vi "W&R(Know Size Without Check With Data).vi"(0 "VISA resource name in":refnum<visa-resource-name>, 5 "写入指令/数据":string, 7 "总字节数":u32, 9 "超时":u32=1000, 11 "error in":errorcluster) -> (4 "VISA resource name out":refnum<visa-resource-name>, 6 "读取缓冲区":string, 15 "error out":errorcluster)   [LabVIEW 2020]
uses:
  <vilib>/Instr/_visa.llb/VISA Set IO Buffer Mask.ctl
  <vilib>/Instr/_visa.llb/VISA Flush IO Buffer Mask.ctl
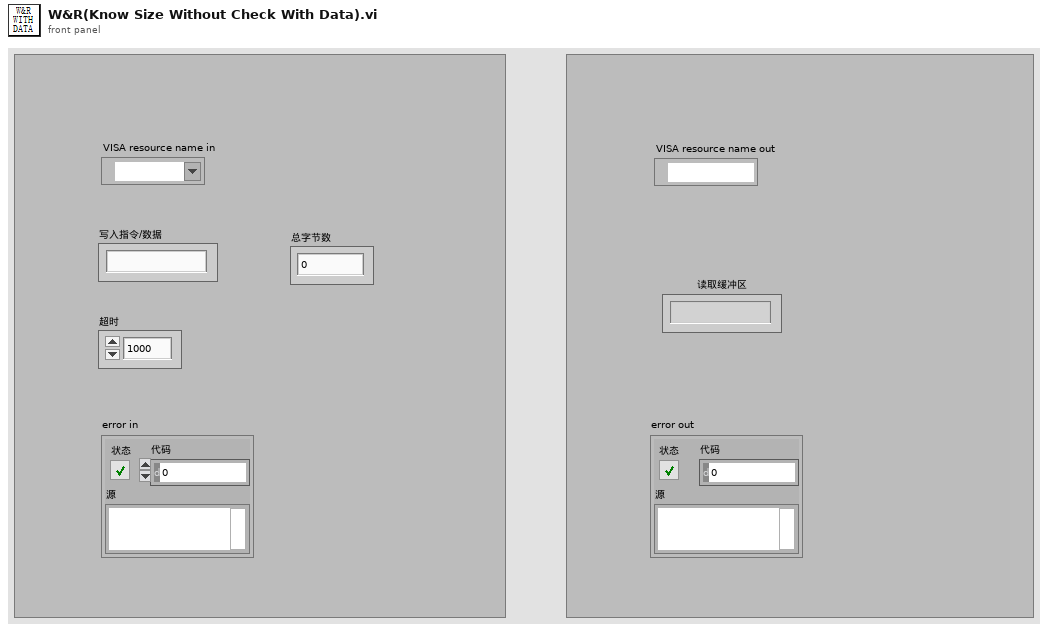
[diagram p1: front panel]
types:
  T1 = typedef "VISA Flush IO Buffer Mask.ctl" = u16
  T2 = typedef "VISA Set IO Buffer Mask.ctl" = u16
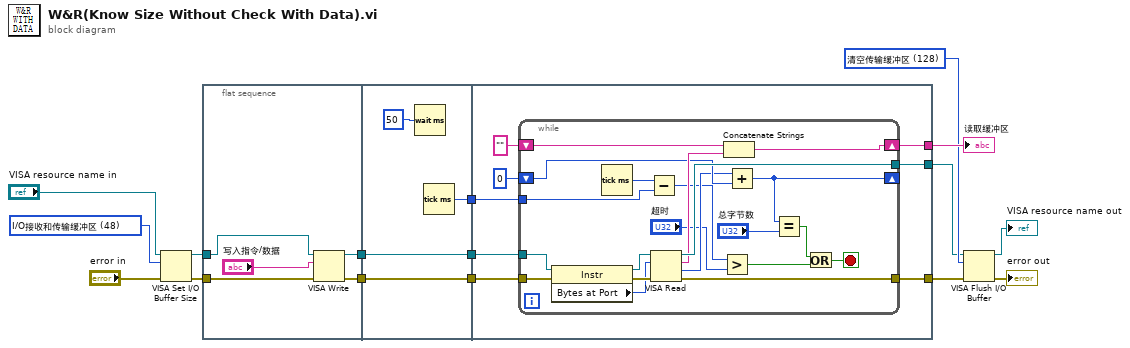
[diagram p0: block diagram]
diagram:
  w9 = T1 128 items=["清空接收缓冲区"=16, "向设备写入传输缓冲区"=32, "清空接收缓冲区（无I/O）"=64, "清空传输缓冲区"=128] ("Mask")
  w10 = T2 48 items=["I/O接收缓冲区"=16, "I/O传输缓冲区"=32, "I/O接收和传输缓冲区"=48] ("Mask")
  n1 = VISA Set I/O Buffer Size(VISA resource name="VISA resource name in", mask (16)=w10, error in (no error)="error in") -> (VISA resource name out=w6:refnum<visa-resource-name>, error out=w5:errorcluster)  [unwired: 1 in]
  n2 = flat-sequence {
    tunnel: w6 -> [w21]
    tunnel: [w20] -> w16
    tunnel: [w18] -> w15
    tunnel: w5 -> [w17]
    tunnel: [w25] -> w14
    tunnel: w16 -> [w25]
    tunnel: [w24] -> w13
    tunnel: w15 -> [w24]
    tunnel: [w23] -> w12
    tunnel: w14 -> [w33]
    tunnel: w13 -> [w32]
    tunnel: [w31] -> w4
    tunnel: [w30] -> w3
    tunnel: w12 -> [w27]
    tunnel: [w26] -> w11
    frame #0 {
      n3 = VISA Write(VISA resource name=w21, write buffer="写入指令/数据", error in (no error)=w17) -> (VISA resource name out=w20:refnum<visa-resource-name>, error out=w18:errorcluster)  [unwired: 1 out]
    }
    frame #1 {
      n4 = Wait (ms)(milliseconds to wait=u32 50 ("等待时间（毫秒）")) -> ()  [unwired: 1 out]
      n5 = Tick Count (ms)() -> (millisecond timer value=w23:u32)
    }
    frame #2 {
      n6 = while {
        tunnel: w33 -> [w54]
        tunnel: w32 -> [w53]
        shift-right: [w50] -> w26
        shift-left: "" -> [w49]
        tunnel: [w48] -> w31
        tunnel: [w47] -> w30
        shift-right: [w43] -> _
        shift-left: u32 0 -> [w44]
        tunnel: w27 -> [w39]
        stop <- w35 stop-if-true
        n7 = property class="Instr"(reference=w54, error in=w53) -> (reference out=w52:refnum<visa-resource-name>, error out=w51:errorcluster, "Bytes at Port"=w45:u32)
        n8 = Tick Count (ms)() -> (millisecond timer value=w40:u32)
        n9 = Subtract(x=w40, y=w39) -> (x-y=w38:u32)
        n10 = VISA Read(VISA resource name=w52, byte count=w45, error in (no error)=w51) -> (VISA resource name out=w48:refnum<visa-resource-name>, read buffer=w46:string, return count=w41:u32, error out=w47:errorcluster)
        n11 = Greater?(x=w38, y="超时") -> (0:w36:bool)
        n12 = Concatenate Strings(w49, w46) -> (w50:string)
        n13 = Add(x=w41, y=w44) -> (x+y=w43:u32)
        n14 = Equal?(x=w43, y="总字节数") -> (x = y?=w37:bool)
        n15 = Or(x=w37, y=w36) -> (x .or. y?=w35:bool)
      }
    }
  }
  n16 = VISA Flush I/O Buffer(VISA resource name=w4, mask (16)=w9, error in (no error)=w3) -> (VISA resource name out=→"VISA resource name out":refnum<visa-resource-name>, error out=→"error out":errorcluster)
  "读取缓冲区" <- w11
